vi "DriveTrain Control.vi"(10 "Left Drive In":dbl, 11 "Right Drive In":dbl) -> (2 "Left Drive Out":dbl, 3 "Right Drive Out":dbl)   [LabVIEW 2015]
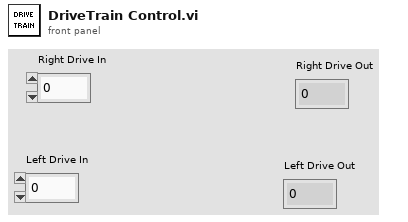
[diagram p1: front panel]
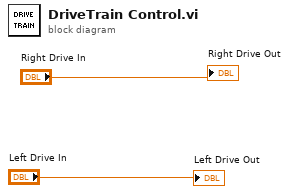
[diagram p0: block diagram]
diagram:
  "Right Drive Out" <- "Right Drive In"
  "Left Drive Out" <- "Left Drive In"
